vi "RandI32.vi"(3 "Limit b":i32=1 caption="Limit b (1)", 5 "Limit a":i32 caption="Limit a (0)") -> (1 "Random number":i32)   [LabVIEW 2017, in "GPNumeric.lvlib"]
doc: "Produces a <B>Random number</B> between <B>Limit a</B> and <B>Limit b</B>.\n\nIt doesn't matter which of <B>Limit a</B> and <B>Limit b</B> is highest, only the range is considered. Both limits are included in the range of random numbers.\n\nThis VI is polymorphic, right click on it to select the data type.\n\nThis VI is inlined.\n\nSteen Schmidt\nGPower\n5/4 2014"
uses:
  GPNumeric.lvlib
panel:
  # "Copyright © 2014\nGPower\nSee enclosed license file for terms and conditions"
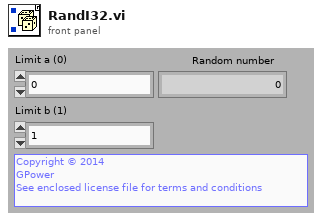
[diagram p1: front panel]
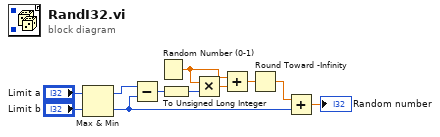
[diagram p0: block diagram]
diagram:
  n1 = Max & Min(x="Limit a", y="Limit b") -> (max(x,y)=w7:i32, min(x,y)=w6:i32)
  n2 = Subtract(x=w7, y=w6) -> (x-y=w5:i32)
  n3 = Random Number (0-1)() -> (number: 0 to 1=w1:dbl)
  n4 = To Unsigned Long Integer(number=w5) -> (unsigned 32bit integer=w4:u32)
  n5 = Multiply(x=w1, y=w4) -> (x*y=w3:dbl)
  n6 = Add(x=w1, y=w3) -> (x+y=w2:dbl)
  n7 = Round Toward -Infinity(1:w2) -> (0:w8:dbl)
  n8 = Add(x=w8, y=w6) -> (x+y=→"Random number":dbl)
